vi "InsideObstruction.vi"(8 "error in (no error)":errorcluster, 10 "point":cluster{"X":dbl, "Y":dbl}, 11 "Obstruction in":refnum<class "Obstruction.lvclass">) -> (0 "error out":errorcluster, 2 "inside":bool, 3 "Obstruction out":refnum<class "Obstruction.lvclass">)   [LabVIEW 2013, in "Obstruction.lvclass"]
uses:
  Obstruction.lvclass
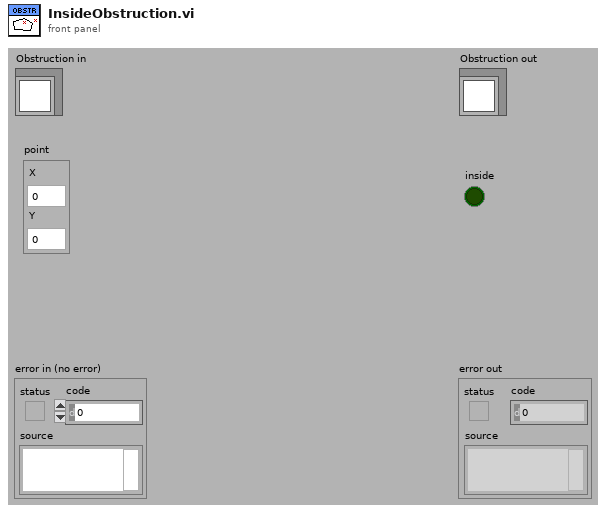
[diagram p1: front panel]
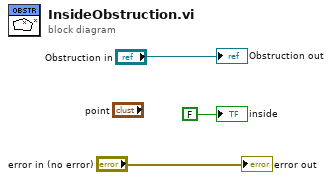
[diagram p0: block diagram]
diagram:
  "error out" <- "error in (no error)"
  "Obstruction out" <- "Obstruction in"
  "inside" <- FALSE ("inside")
